vi "CLD 2  Elapsed Time Express with pause Front Panel.vi"() -> ()   [LabVIEW 2009]
doc: "CLD 2, Challenge Exercise"
panel:
  out "Elapsed Time (s)":dbl
  out "Time Has Elapsed":bool
  in  "Auto Reset":bool
  in  "Pause Button":bool
  in  "Reset Button":bool
  in  "Stop VI":bool
  out "error out":errorcluster
  in  "error in (no error)":errorcluster
  in  "Time Target (s)":dbl
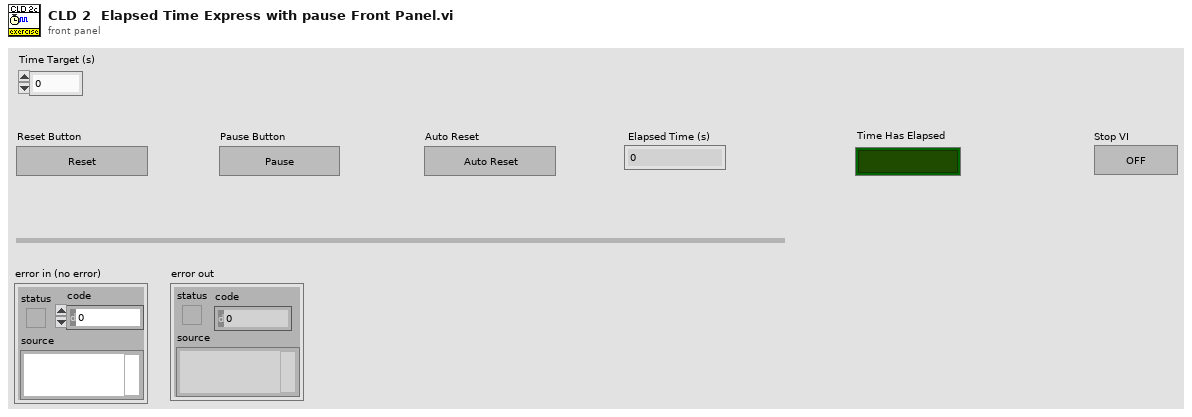
[diagram p1: front panel]
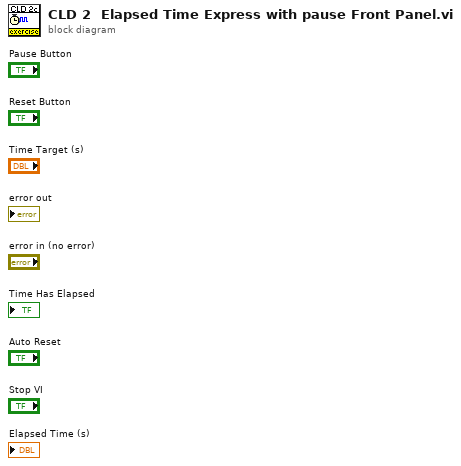
[diagram p0: block diagram]
diagram:
